vi "Get Project Scan Path.vi"(11 "Test Project Path":path) -> (1 "Framework Path":path, 2 "IsFramework":bool, 3 "Test Project Scan Path":path)   [LabVIEW 2011, in "VITesterUtilities.lvlib"]
uses:
  Libraries/VITesterUtilities.lvlib
  <userlib>/_OpenG.lib/file/file.llb/Strip Path Extension - Path__ogtk.vi
  <userlib>/_OpenG.lib/file/file.llb/Strip Path - Traditional__ogtk.vi
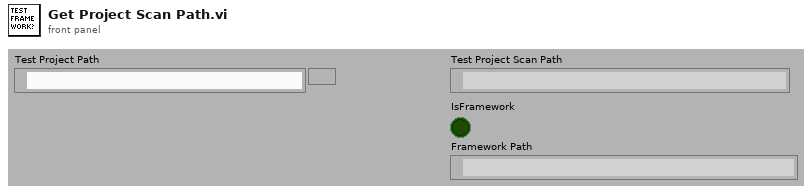
[diagram p1: front panel]
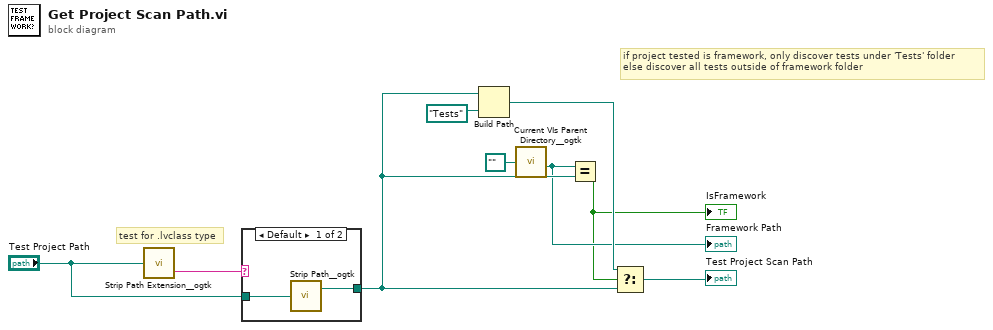
[diagram p0: block diagram]
diagram:
  # "if project tested is framework, only discover tests under 'Tests' folder\nelse discover all tests outside of framework folder"
  # "test for .lvclass type"
  n1 = call-poly <userlib>:"Strip Path Extension__ogtk.vi"("path"="Test Project Path") -> ("extension"=w2:string)  [unwired: 1 out]
  n2 = case shown="Default" w2 {
    tunnel: "Test Project Path" -> [w11 w12]
    tunnel: [w10 w12] -> w9
    frame Default {
      n3 = call-poly <userlib>:"Strip Path__ogtk.vi"("path"=w11) -> ("stripped path"=w10:path)  [unwired: 1 out]
    }
    frame "" {
    }
  }
  n4 = Build Path(base path=w9, name or relative path=path "Tests" ("Relative path (.)")) -> (appended path=w7:path)
  n5 = call <userlib>:"Current VIs Parent Directory__ogtk.vi"("Relative path (.)"=path "..") -> ("Parent Directory (+ Relative)"=w5:path)  [unwired: 4 in]
  "Framework Path" <- w5
  n6 = Equal?(x=w5, y=w9) -> (x = y?=w1:bool)
  "IsFramework" <- w1
  n7 = Select(t=w7, s=w1, f=w9) -> (s? t:f=→"Test Project Scan Path":path)
